vi "Create.vi"(4 "TypeMap in":refnum<class "TypeMap.lvclass">, 6 "commandTimeout":i32=-1, 8 "error in (no error)":errorcluster, 10 "object in":refnum<class>, 11 "SqlMapper in":refnum<class "SqlMapper.lvclass">) -> (0 "error out":errorcluster, 1 "id":i32, 2 "object out":refnum<class>, 3 "SqlMapper out":refnum<class "SqlMapper.lvclass">)   [LabVIEW 2020, in "ORM.lvlib" / "TypeMap.lvclass"]
uses:
  TypeMap.lvclass
  SqlMapper/SqlMapper.lvclass
  TypeMap.lvclass/TypeMap.ctl
  Read Autokey.vi
  Read Table Name.vi
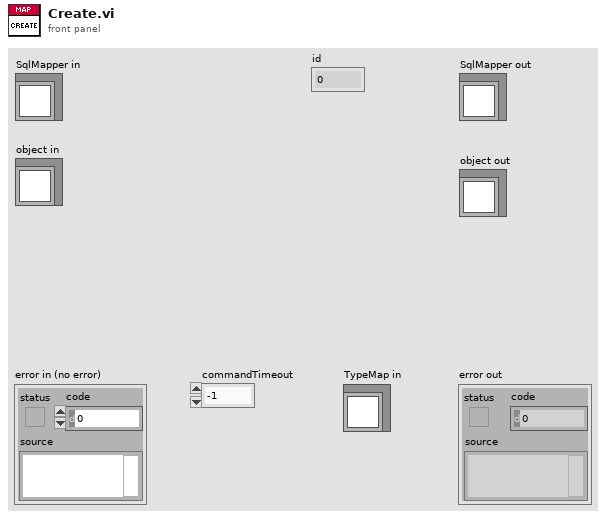
[diagram p1: front panel]
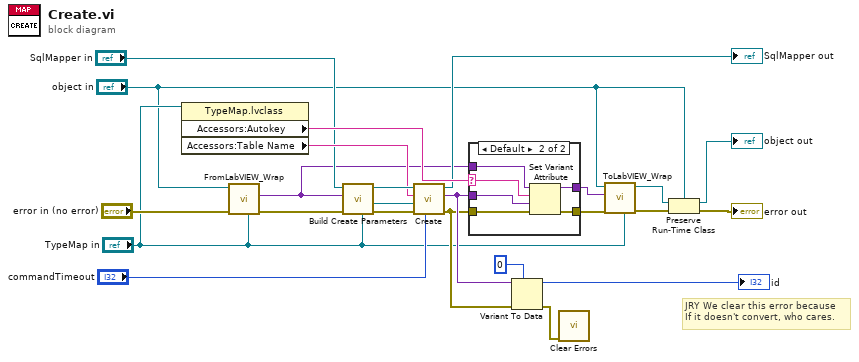
[diagram p0: block diagram]
diagram:
  # "JRY We clear this error because\nIf it doesn't convert, who cares."
  n1 = property class="TypeMap.lvclass"(reference="TypeMap in") -> ("Accessors:Autokey"=w16:string, "Accessors:Table Name"=w10:string)  [unwired: 1 in, 2 out]
  n2 = call "FromLabVIEW_Wrap.vi"("TypeMap in"="TypeMap in", "error in (no error)"="error in (no error)", "object in"="object in") -> ("error out"=w24:errorcluster, "DbRow"=w4:variant)  [unwired: 7 in]
  n3 = call-dynamic "Build Create Parameters.vi"("TypeMap in"="TypeMap in", "error in (no error)"=w24, "object"=w4, "SqlMapper in"="SqlMapper in") -> ("error out"=w22:errorcluster, "DynamicParameters out"=w21:refnum<class "DynamicParameters.lvclass">, "SqlMapper out"=w23:refnum<class "SqlMapper.lvclass">)  [unwired: 5 in]
  n4 = call "Create.vi"("commandTimeout"="commandTimeout", "error in (no error)"=w22, "DynamicParameters"=w21, "tableName"=w10, "SqlMapper in"=w23) -> ("error out"=w14:errorcluster, "id"=w15:variant, "SqlMapper out"=→"SqlMapper out":refnum<class "SqlMapper.lvclass">)  [unwired: 4 in]
  n5 = case shown="Default" w16 {
    selector: w16 -> [_ w30]
    tunnel: [w26 w32] -> w17
    tunnel: w4 -> [w25 w31]
    tunnel: w14 -> [w26 w27]
    tunnel: w15 -> [_ w28]
    tunnel: [w25 w29] -> w1
    frame "" {
    }
    frame Default {
      n6 = Set Variant Attribute(Variant=w31, name=w30, value=w28, error in=w27) -> (Variant out=w29:variant, error out=w32:errorcluster)  [unwired: 1 out]
    }
  }
  n7 = Variant To Data(error in=w14, type=0, Variant=w15) -> (data=→"id":i32, error out=w11:errorcluster)
  n8 = call <vilib>:"Clear Errors.vi"("error in (no error)"=w11) -> ()  [unwired: 5 in, 2 out]
  n9 = call "ToLabVIEW_Wrap.vi"("TypeMap in"="TypeMap in", "error in (no error)"=w17, "DbRow"=w1, "TargetObject In"="object in") -> ("error out"=w18:errorcluster, "Object Out"=w6:refnum<class>)  [unwired: 6 in]
  n10 = Preserve Run-Time Class(object in=w6, error in=w18, 2:"object in") -> (object out=→"object out":refnum<class>, error out=→"error out":errorcluster)
